vi "Modbus.ReadCoils.vi"(8 "error in (no error)":errorcluster, 11 "address":T1) -> (0 "error out":errorcluster, 2 "data":bool[](array[boolean]), 3 "Coils":i16[](array[numeric]))   [LabVIEW 2019, in "Modbus.lvlib"]
uses:
  Modbus.lvlib
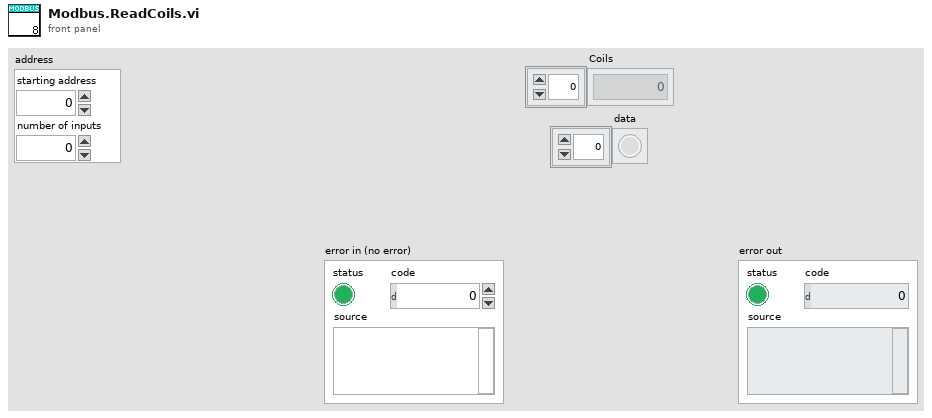
[diagram p1: front panel]
types:
  T1 = cluster{"starting address":u16, "number of inputs":u16}
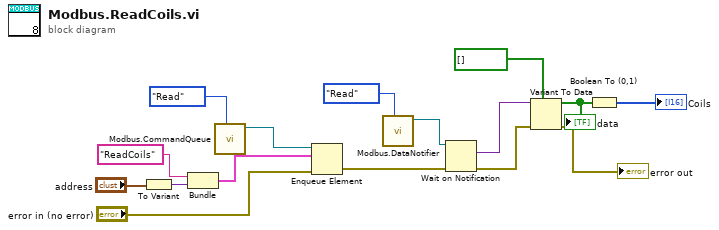
[diagram p0: block diagram]
diagram:
  n1 = To Variant(anything="address") -> (Variant=w12:variant)
  n2 = Bundle("ReadCoils", "Variant"=w12) -> (w13:cluster{string, "Variant":variant})  [unwired: 1 in]
  n3 = call "Modbus.CommandQueue.vi"("OP"=enum16{"Read", "Write"}."Read") -> ("queue OUT"=w15:refnum<queue>)  [unwired: 10 in]
  n4 = Enqueue Element(queue=w15, element=w13, error in (no error)="error in (no error)") -> (error out=w8:errorcluster)  [unwired: 1 in, 2 out]
  n5 = call "Modbus.DataNotifier.vi"("OP"=enum16{"Read", "Write"}."Read") -> ("notifier OUT"=w7:refnum<notifier>)  [unwired: 10 in]
  n6 = Wait on Notification(notifier=w7, error in (no error)=w8) -> (notification=w6:variant, error out=w4:errorcluster)  [unwired: 2 in, 2 out]
  n7 = Variant To Data(error in=w4, type=bool[] [], Variant=w6) -> (data=w2:bool[], error out=→"error out":errorcluster)
  "data" <- w2
  n8 = Boolean To (0,1)(Boolean=w2) -> (0, 1=→"Coils":i16[])
